vi "FGV_BufferUsageMetrics.vi"(7 "?":T1, 11 "Input":dbl format="%#_13g") -> (2 "MIDAS Buffer Usage (%)":dbl(knob) scale=0.0..100.0, 3 "DataPacker Queue Usage (%)":dbl(knob) scale=0.0..100.0)   [LabVIEW 2018, in "feGEM DataPacker.lvlib"]
uses:
  feGEM DataPacker.lvlib
  DataPacker_Buffer_Usage_Enum.ctl
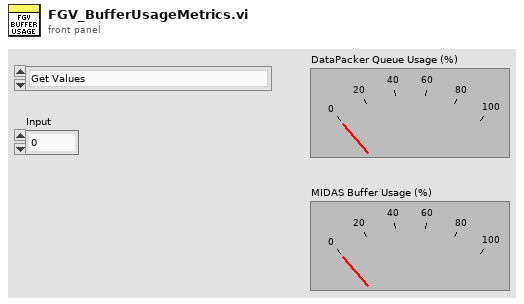
[diagram p1: front panel]
types:
  T1 = typedef "feGEM DataPacker.lvlib/DataPacker_Buffer_Usage_Enum.ctl" = enum16{"Get Values", "Set MIDAS Buffer Usage (%)", "Set DataPacker Queue\nUsage (%)"}
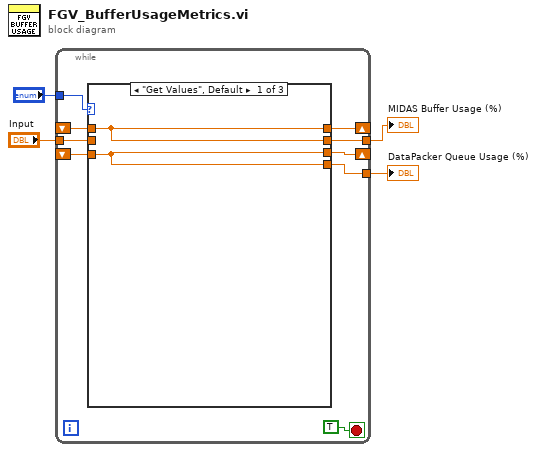
[diagram p0: block diagram]
diagram:
  n1 = while {
    tunnel: "Input" -> [w11]
    tunnel: "?" -> [w12]
    tunnel: [w10] -> w2
    shift-right: [w9] -> _
    shift-left: _ -> [w7]
    shift-right: [w8] -> _
    shift-left: _ -> [w6]
    tunnel: [w5] -> w1
    stop <- TRUE stop-if-true
    n2 = case shown="\"Get Values\", Default" w12 {
      tunnel: w11 -> [_ w17 w19]
      tunnel: [w14 w16 w19] -> w10
      tunnel: [w15 w17 w18] -> w9
      tunnel: [w14 w16 w19] -> w8
      tunnel: w7 -> [w15 _ w18]
      tunnel: w6 -> [w14 w16 _]
      tunnel: [w15 w17 w18] -> w5
      frame "Get Values", Default {
      }
      frame "Set MIDAS Buffer Usage (%)" {
      }
      frame "Set DataPacker Queue\nUsage (%)" {
      }
    }
  }
  "DataPacker Queue Usage (%)" <- w2
  "MIDAS Buffer Usage (%)" <- w1
